vi "UHR-Fleezers Control (host) -Leonardo 04-2018 V3.vi"(0 "Tab Control":T5(tab)=enum."Trap Control (RF)") -> ()   [LabVIEW 2013] (continued)
              tunnel: w2124 -> [w2130]
              tunnel: w2122 -> [w2129]
              tunnel: w2121 -> [w2128]
              tunnel: w2120 -> [w2127]
              stop <- w2132 stop-if-true
              n1371 = event shown="[0] \"Pane\": Mouse Move" {
                selector: _ -> [_ _]
                dyn-events: _ -> [_ _]
                timeout: _ -> [_ _]
                tunnel: ["Force Manip Abort" w2196] -> w2132
                tunnel: w2131 -> [w2139 _]
                tunnel: w2130 -> [w2137 _]
                tunnel: w2129 -> [w2136 _]
                tunnel: w2128 -> [w2135 _]
                tunnel: w2127 -> [w2134 _]
                event Mouse Move {
                  n1372 = event-data() -> ("Time"=w2140:u32, "Coords"=w2141:T8)  [unwired: 3 out]
                  n1373 = Less?(x=w2140, y=w2139) -> (x < y?=w2138:bool)
                  n1374 = case "Makes sure old motion events prior to mouse click aren't used" shown="False" w2138 {
                    tunnel: w2141 -> [w2183 _]
                    tunnel: w2137 -> [w2184 _]
                    tunnel: w2136 -> [w2161 _]
                    tunnel: w2135 -> [w2157 _]
                    tunnel: w2134 -> [w2156 _]
                    frame False {
                      n1375 = Subtract(x=w2183, y=w2184) -> (x-y=w2182:T8)
                      "Coords" <- w2182
                      n1376 = local read "Y RF Frequency Limits (MHz)"() -> (w2142:T16)
                      n1377 = To Double Precision Float(number=w2182) -> (double precision float=w2181:cluster{"Horizontal":dbl, "Vertical":dbl})
                      n1378 = Multiply(x=cluster{"Horizontal":dbl, "Vertical":dbl} {"Horizontal"=-1.0, "Vertical"=1.0}, y="Manipulation Scaling") -> (x*y=w2177:cluster{"Horizontal":dbl, "Vertical":dbl})
                      n1379 = local read "X RF Frequency Limits (MHz)"() -> (w2143:T16)
                      n1380 = Multiply(x=w2181, y=w2177) -> (x*y=w2179:cluster{"Horizontal":dbl, "Vertical":dbl})
                      n1381 = Unbundle By Name(w2179) -> ("Horizontal"=w2174:dbl, "Vertical"=w2178:dbl)
                      n1382 = Unbundle By Name(w2142) -> ("Maximum"=w2145:dbl, "Minimum"=w2144:dbl)
                      n1383 = Boolean To (0,1)(Boolean="Manip. X?") -> (0, 1=w2172:i16)
                      n1384 = Boolean To (0,1)(Boolean="Manip. Y?") -> (0, 1=w2169:i16)
                      n1385 = local read "BD 1 Frequency 2 (MHz)"() -> (w2159:dbl)
                      n1386 = Multiply(x=w2178, y=w2169) -> (x*y=w2171:dbl)
                      n1387 = Multiply(x=w2172, y=w2174) -> (x*y=w2175:dbl)
                      n1388 = local read "BD 2 Frequency 2 (MHz)"() -> (w2158:dbl)
                      n1389 = Unbundle By Name(w2143) -> ("Maximum"=w2147:dbl, "Minimum"=w2146:dbl)
                      n1390 = Add(x=w2156, y=w2171) -> (x+y=w2149:dbl)
                      n1391 = Add(x=w2157, y=w2175) -> (x+y=w2151:dbl)
                      n1392 = In Range and Coerce(upper limit=w2147, x=w2151, lower limit=w2146) -> (coerced(x)=w2150:dbl)  [unwired: 1 out]
                      n1393 = In Range and Coerce(upper limit=w2145, x=w2149, lower limit=w2144) -> (coerced(x)=w2148:dbl)  [unwired: 1 out]
                      n1394 = Subtract(x=w2150, y=w2159) -> (x-y=w2168:dbl)
                      n1395 = Subtract(x=w2148, y=w2158) -> (x-y=w2167:dbl)
                      n1396 = Square(x=w2168) -> (x^2=w2166:dbl)
                      n1397 = Square(x=w2167) -> (x^2=w2165:dbl)
                      n1398 = Add(x=w2166, y=w2165) -> (x+y=w2164:dbl)
                      n1399 = Square Root(x=w2164) -> (sqrt(x)=w2160:dbl)
                      n1400 = In Range and Coerce(upper limit="Limit Max (MHz)", x=w2160, lower limit="Limit Min (MHz)") -> (In Range?=w2153:bool)  [unwired: 1 out]
                      n1401 = Not(x="Limits Enable") -> (.not. x?=w2152:bool)
                      n1402 = Or(x=w2153, y=w2152) -> (x .or. y?=w2154:bool)
                      n1403 = case shown="True" w2154 {
                        tunnel: w2161 -> [_ w2194]
                        tunnel: w2160 -> [_ w2185]
                        tunnel: w2150 -> [_ w2192]
                        tunnel: w2159 -> [_ w2191]
                        tunnel: w2148 -> [_ w2190]
                        tunnel: w2158 -> [_ w2189]
                        tunnel: w2143 -> [_ w2187]
                        tunnel: w2142 -> [_ w2186]
                        frame False {
                        }
                        frame True {
                          n1404 = local read "BD 1 Frequency 3 (MHz)"() -> (w2193:dbl)
                          n1405 = local read "BD 2 Frequency 3 (MHz)"() -> (w2188:dbl)
                          n1406 = local write "Trap Delta (MHz)"(w2185) -> ()
                          n1407 = property on="Initial delta (MHz)" class="DigNum (strict)"("Val(Sgnl)"=w2185) -> ()  [unwired: 2 in, 2 out]
                          n1408 = call "set RF board frequency - interlace.vi"("Board 2 Frequency Limits"=w2186, "Board 1 Frequency Limits"=w2187, "FPGA VI Reference In"=w2194, "Board 2 Frequency 3 (MHz)"=w2188, "Board 1 Frequency 3 (MHz)"=w2193, "Board 2 Frequency 2 (MHz)"=w2189, "Board 2 Frequency 1 (MHz)"=w2190, "Board 1 Frequency 2 (MHz)"=w2191, "Board 1 Frequency 1  (MHz)"=w2192) -> ()  [unwired: 1 in, 2 out]
                          n1409 = local write "BD 2 Frequency 1 (MHz)"(w2190) -> ()
                          n1410 = local write "BD 1 Frequency 1 (MHz)"(w2192) -> ()
                        }
                      }
                    }
                    frame True {
                    }
                  }
                }
                event Mouse Up {
                  n1411 = event-data() -> ("Button"=w2195:u16)  [unwired: 8 out]
                  n1412 = case shown="3" w2195 {
                    tunnel: [FALSE TRUE] -> w2196
                    frame 0, Default {
                    }
                    frame 3 {
                      n1413 = local write "Manipulating Trap"(FALSE ("Manipulating Trap")) -> ()
                    }
                  }
                }
              }
            }
          }
        }
      }
      event Mouse Move {
        n1414 = event-data() -> ()  [unwired: 6 out]
      }
    }
    n1415 = local read "Stop All"() -> (w2017:bool)
    n1416 = node-c288() -> ()  [unwired: 2 out]
  }
  n1417 = node-c288(w49) -> ()  [unwired: 1 out]
  n1418 = node-c288(w101) -> ()  [unwired: 1 out]
  n1419 = node-c288(w108) -> ()  [unwired: 1 out]
  n1420 = node-c288(i64 1 ("Period"), 1 ("Processor")) -> (w194:T25)  [unwired: 2 out]
  n1421 = timed-loop "Acquire Data" {
    tunnel: w57 -> [w2505]
    tunnel: w73 -> [w2504]
    tunnel: [w2535] -> w66
    tunnel: [w2529] -> w65
    timing: w194 -> [_]
    timing-out: [_] -> w193
    tunnel: w92 -> [w2351]
    stop <- "Stop All" stop-if-true
    (unwired) u32 0 ("Number of Elements")
    w2338 = "NI_ChannelName" ("name")
    n1422 = node-c288() -> ()  [unwired: 2 out]
    n1423 = First Call?() -> (First Call?: T/F=w2304:bool)
    n1424 = Or(x="Reset", y=w2304) -> (x .or. y?=w2305:bool)
    n1425 = local read "MCL Tracking"() -> (w2242:bool)
    n1426 = case "Reset data stream" shown="True" w2305 {
      tunnel: w2505 -> [w2655 w2663]
      tunnel: w2504 -> [w2654 w2662]
      tunnel: [w2655 w2657] -> w2240
      tunnel: [w2654 w2656] -> w2500
      frame False {
      }
      frame True {
        w2660 = TRUE ("AI to FIFO")
        n1427 = local write "Overflow (data lost)"(FALSE ("Overflow (data lost)")) -> ()
        n1428 = call "reset FPGA DMA.vi"("error in"=w2662, "FPGA VI Reference In"=w2663) -> ("error out"=w2658:errorcluster, "FPGA VI Reference Out"=w2659:T20)
        n1429 = xnode "Read/Write Control"("FPGA VI Reference In"=w2659, "error in"=w2658, "AI to FIFO"=w2660, "APD to FIFO"=w2660) -> ("FPGA VI Reference Out"=w2657:T20, "error out"=w2656:errorcluster)
      }
    }
    n1430 = Or(x="Start AOD Scan", y="Trap Raster Scan") -> (x .or. y?=w2458:bool)
    n1431 = case "Start AOM raster scan" shown="True" w2458 {
      tunnel: w2240 -> [w3396 w3407]
      tunnel: w2500 -> [w3395 w3406]
      tunnel: [w3396 w3400] -> w2239
      tunnel: [w3395 w3399] -> w2499
      frame False {
      }
      frame True {
        n1432 = case shown="True" "Restart DMA? (AOD)" {
          tunnel: [w3447 w3449] -> w3401
          tunnel: [w3446 w3448] -> w3402
          tunnel: w3407 -> [w3447 w3451]
          tunnel: w3406 -> [w3446 w3450]
          frame False {
          }
          frame True {
            n1433 = local write "Overflow (data lost)"(FALSE ("Overflow (data lost)")) -> ()
            n1434 = call "reset FPGA DMA.vi"("error in"=w3450, "FPGA VI Reference In"=w3451) -> ("error out"=w3448:errorcluster, "FPGA VI Reference Out"=w3449:T20)
          }
        }
        n1435 = local write "Trap Raster Scan"(FALSE ("Trap Raster Scan")) -> ()
        n1436 = case shown="True" "Move MCL Also?" {
          tunnel: w3402 -> [w3411 w3441]
          tunnel: w3401 -> [w3412 w3442]
          tunnel: [w3410 w3445] -> w3400
          tunnel: [w3409 w3444] -> w3399
          tunnel: "Raster to target force?" -> [w3408 w3414]
          frame False {
            w3413 = TRUE ("AI to FIFO")
            n1437 = xnode "Read/Write Control"("FPGA VI Reference In"=w3412, "error in"=w3411, "AI to FIFO"=w3413, "APD to FIFO"=w3413, "Start scan"=w3413, "Raster to target force"=w3408) -> ("FPGA VI Reference Out"=w3410:T20, "error out"=w3409:errorcluster)
          }
          frame True {
            w3438 = FALSE ("1D or 2D Scan?")
            w3443 = TRUE ("AI to FIFO")
            # "Count for MCL loop"
            # "N total cycles"
            # "N steps"
            # "V_int"
            n1438 = local read "Scan Range (nm)"() -> (w3420:dbl)
            n1439 = local read "Number of F/B Scans (AOD)"() -> (w3437:u16)
            n1440 = Sign(1:w3420) -> (0:w3419:dbl)
            n1441 = Compound Arithmetic op=MULTIPLY(w3420, "MCL Step Position Ratio", "MCL/AOM Scale Tweak") -> (w3424:dbl)
            n1442 = Negate(x=w3419) -> (-x=w3416:dbl)
            n1443 = Multiply(x=w3416, y="MCL Step Increment (V_int)") -> (x*y=w3418:dbl)
            n1444 = Divide(x=w3424, y="MCL X Cal (nm/V)") -> (x/y=w3430:dbl)
            n1445 = Multiply(x=32767.0 ("y"), y=w3430) -> (x*y=w3436:dbl)
            n1446 = local read "Total Counts (ticks)"() -> (w3421:u32)
            n1447 = local read "Cycles/step (AOD)"() -> (w3432:u64)
            n1448 = local read "Scan steps (AOD)"() -> (w3433:u64)
            n1449 = Divide(x=w3436, y=10.0) -> (x/y=w3429:dbl)
            n1450 = Divide(x=w3429, y="MCL Step Increment (V_int)") -> (x/y=w3427:dbl)
            n1451 = Absolute Value(x=w3427) -> (abs(x)=w3415:dbl)
            n1452 = Compound Arithmetic op=MULTIPLY(w3433, w3432, w3421) -> (w3428:u64)
            n1453 = local write "wait to reset values"(w3443) -> ()
            n1454 = local write "MCL Scanning"(w3443) -> ()
            n1455 = Divide(x=w3428, y=w3415) -> (x/y=w3425:dbl)
            "MCL Count" <- w3425
            n1456 = xnode "Read/Write Control"("FPGA VI Reference In"=w3442, "error in"=w3441, "Scan steps (MCL)"=w3415, "Number of scans (MCL)"=w3437, "Cycles per step (MCL)"=u64 1, "Scan freq.  increment (MCL)"=w3418, "1D or 2D Scan?"=w3438, "MCL Scan Axis"=w3438, "Cont. Scan (MCL)"=w3438, "MCL count"=w3425) -> ("FPGA VI Reference Out"=w3440:T20, "error out"=w3439:errorcluster)
            n1457 = xnode "Read/Write Control"("FPGA VI Reference In"=w3440, "error in"=w3439, "AI to FIFO"=w3443, "APD to FIFO"=w3443, "Start scan"=w3443, "Start scan (MCL)"=w3443, "Raster to target force"=w3414) -> ("FPGA VI Reference Out"=w3445:T20, "error out"=w3444:errorcluster)
          }
        }
        "Raster Scanning..." <- TRUE ("Scanning...")
      }
    }
    n1458 = And(x="Save scans", y=w2458) -> (x .and. y?=w2498:bool)
    n1459 = Compound Arithmetic op=OR("Start MCL Scan", "Confocal Image", "Confocal Linescan") -> (w2456:bool)
    n1460 = And(x="Save Data (MCL)", y=w2456) -> (x .and. y?=w2497:bool)
    n1461 = case "Start MCL raster scan" shown="True" w2456 {
      tunnel: w2239 -> [w2946 w2961]
      tunnel: w2499 -> [w2945 w2960]
      tunnel: [w2946 w2956] -> w2274
      tunnel: [w2945 w2955] -> w2273
      tunnel: [FALSE w2954] -> w2483
      tunnel: "Start MCL Scan" -> [_ w2949]
      tunnel: "Confocal Image" -> [_ w2948]
      tunnel: "Confocal Linescan" -> [_ _]
      frame False {
      }
      frame True {
        w2954 = TRUE
        n1462 = case shown="True" "Restart DMA? (MCL)" {
          tunnel: [w3006 w3008] -> w2959
          tunnel: [w3005 w3007] -> w2958
          tunnel: w2961 -> [w3006 w3011]
          tunnel: w2960 -> [w3005 w3010]
          frame False {
          }
          frame True {
            n1463 = call "reset FPGA DMA.vi"("error in"=w3010, "FPGA VI Reference In"=w3011) -> ("error out"=w3007:errorcluster, "FPGA VI Reference Out"=w3008:T20)
            n1464 = local write "Overflow (data lost)"(FALSE ("Overflow (data lost)")) -> ()
          }
        }
        n1465 = case shown="False" w2949 {
          selector: w2949 -> [_ w2965]
          tunnel: w2948 -> [w2964 _]
          tunnel: [w2964 w2965] -> w2947
          frame False {
            n1466 = property on="2D or 1D Scan" class="Bool (strict)"("Val(Sgnl)"=w2964) -> ()  [unwired: 2 in, 2 out]
            n1467 = property on="Confocal Image" class="Bool (strict)"("Value"=FALSE ("Start Confocal Map")) -> ()  [unwired: 2 in, 2 out]
          }
          frame True {
          }
        }
        n1468 = local write "MCL Scanning"(w2954) -> ()
        n1469 = local read "AO1"() -> (w2951:dbl)
        n1470 = local read "AO2"() -> (w2950:dbl)
        n1471 = case shown="True" "Center Scan" {
          tunnel: w2959 -> [w2972 w3004]
          tunnel: w2958 -> [w2971 w3003]
          tunnel: [w2970 w3002] -> w2956
          tunnel: [w2969 w3001] -> w2955
          tunnel: [w2967 w2988] -> w2953
          tunnel: [w2966 w2987] -> w2952
          tunnel: w2951 -> [w2967 w2993]
          tunnel: w2950 -> [w2966 w2996]
          tunnel: w2947 -> [_ _]
          frame False {
            w2968 = TRUE ("AI to FIFO")
            n1472 = xnode "Read/Write Control"("FPGA VI Reference In"=w2972, "error in"=w2971, "AI to FIFO"=w2968, "APD to FIFO"=w2968, "Start scan (MCL)"=w2968) -> ("FPGA VI Reference Out"=w2970:T20, "error out"=w2969:errorcluster)
          }
          frame True {
            w3000 = TRUE ("AI to FIFO")
            n1473 = local read "Scan steps (MCL)"() -> (w2979:u64)
            n1474 = local read "Scan lines (y)"() -> (w2975:u64)
            n1475 = local read "Fast Scan Dir"() -> (w2986:bool)
            n1476 = local read "Actual MCL Inc (V)"() -> (w2976:dbl)
            n1477 = Decrement(x=w2975) -> (x-1=w2974:u64)
            n1478 = Decrement(x=w2979) -> (x-1=w2978:u64)
            n1479 = Multiply(x=w2976, y=w2974) -> (x*y=w2973:dbl)
            n1480 = Divide(x=w2973, y=2.0) -> (x/y=w2983:dbl)
            n1481 = Multiply(x=w2976, y=w2978) -> (x*y=w2977:dbl)
            n1482 = Divide(x=w2977, y=2.0) -> (x/y=w2982:dbl)
            n1483 = Select(t=w2982, s=w2986, f=w2983) -> (s? t:f=w2981:dbl)
            n1484 = Select(t=w2983, s=w2986, f=w2982) -> (s? t:f=w2985:dbl)
            n1485 = Subtract(x=w2993, y=w2985) -> (x-y=w2984:dbl)
            n1486 = Subtract(x=w2996, y=w2981) -> (x-y=w2980:dbl)
            n1487 = local read "2D or 1D Scan"() -> (w2998:bool)
            n1488 = Not(x=w2986) -> (.not. x?=w2992:bool)
            n1489 = Not(x=w2998) -> (.not. x?=w2994:bool)
            n1490 = And(x=w2986, y=w2994) -> (x .and. y?=w2995:bool)
            n1491 = And(x=w2994, y=w2992) -> (x .and. y?=w2997:bool)
            n1492 = Select(t=w2996, s=w2997, f=w2980) -> (s? t:f=w2987:dbl)
            n1493 = Select(t=w2993, s=w2995, f=w2984) -> (s? t:f=w2988:dbl)
            n1494 = call "Volt to I16.vi"("Voltage In"=w2988) -> ("I16 Voltage Out"=w2991:i16)
            n1495 = call "Volt to I16.vi"("Voltage In"=w2987) -> ("I16 Voltage Out"=w2990:i16)
            n1496 = xnode "Read/Write Control"("FPGA VI Reference In"=w3004, "error in"=w3003, "AI to FIFO"=w3000, "APD to FIFO"=w3000, "Start scan (MCL)"=w3000, "AO1 (Y)"=w2991, "AO2 (X)"=w2990) -> ("FPGA VI Reference Out"=w3002:T20, "error out"=w3001:errorcluster)
          }
        }
        "Initial Y" <- w2953
        "Initial X" <- w2952
        "wait to reset values" <- w2954
      }
    }
    n1497 = local read "Trap Pos Elements/DMA read"() -> (w2347:u32)
    n1498 = local read "Trap AI Elements/DMA read"() -> (w2272:u32)
    n1499 = local read "APD Elements/DMA read"() -> (w2386:u32)
    n1500 = local read "Trap AI FIFO Depth"() -> (w2545:u32)
    n1501 = xnode "Invoke Method"("FPGA VI Reference In"=w2274, "error in"=w2273, "Number of Elements"=w2347, "Timeout (ms)"=-1) -> ("Data"=w2311:u16[], "Elements Remaining"=→"Trap Pos FIFO El Remaining":u32)  [unwired: 2 out]
    n1502 = xnode "Invoke Method"("FPGA VI Reference In"=w2274, "error in"=w2273, "Number of Elements"=w2272, "Timeout (ms)"=-1 ("Timeout")) -> ("FPGA VI Reference Out"=w2243:T20, "error out"=w2275:errorcluster, "Data"=w2271:i16[], "Elements Remaining"=w2276:u32)
    "Trap AI FIFO El. Rem." <- w2276
    n1503 = xnode "Get APD Data"("FPGA VI Reference In"=w2274, "error in"=w2273, "Number of Elements"=w2386, "Timeout (ms)"=-1) -> ("Data"=w2385:u32[], "Elements Remaining"=→"APD FIFO Elements Remaining":u32)  [unwired: 2 out]
    n1504 = Subtract(x=w2545, y=w2272) -> (x-y=w2544:u32)
    n1505 = Decimate 1D Array(w2311) -> (w2308:u16[], w2310:u16[], w2309:u16[])
    n1506 = Divide(x=w2276, y=w2544) -> (x/y=w2543:dbl)
    "Buffer Status" <- w2543
    n1507 = To Unsigned Long Integer(number=w2308) -> (unsigned 32bit integer=w2307:u32[])
    n1508 = Join Numbers(hi=w2310, lo=w2309) -> ((hi.lo)=w2306:u32[])
    n1509 = Equal?(x=w2543, y=1.0) -> (x = y?=w2541:bool)
    n1510 = Join Numbers(hi=w2307, lo=w2306) -> ((hi.lo)=w2300:u64[])
    n1511 = call "IR AOM word to freq - vec.vi"("Frequency Word In (double vec)"=w2300) -> ("Frequency Out"=w2346:dbl[])
    n1512 = case "Alert buffer overflow" shown="True" w2541 {
      frame False {
      }
      frame True {
        n1513 = call <vilib>:"Beep.vi"() -> ()  [unwired: 3 in, 9 out]
        "Overflow (data lost)" <- TRUE ("Overflow (data lost)")
      }
    }
    n1514 = Decimate 1D Array(w2346) -> (w2345:dbl[], w2344:dbl[])
    n1515 = Array Size(array=w2271) -> (size(s)=→"Waveform Chart":i32)
    n1516 = Build Array(w2345, w2344) -> (w2343:dbl[][])
    n1517 = local read "Trap Sets"() -> (w2418:u32)
    n1518 = case "Deinterlace trap data, average down PSD" shown="2" w2418 {
      tunnel: w2271 -> [w3041 w3106]
      tunnel: [w3038 w3103] -> w2411
      tunnel: [w3041 w3105] -> w2303
      tunnel: "Detector Type" -> [w3040 w3101]
      tunnel: [w3039 w3104] -> w2410
      tunnel: [w3037 w3102] -> w2516
      frame 1, Default {
        n1519 = Divide(x=w3041, y=3276.7) -> (x/y=w3042:dbl[])
        n1520 = Decimate 1D Array(w3042) -> (w3051:dbl[], w3050:dbl[], w3049:dbl[], w3048:dbl[], w3047:dbl[], w3046:dbl[], w3045:dbl[], w3044:dbl[])
        n1521 = case shown="\"IR-QPD + PSD + FB-QPD position\"" w3040 {
          tunnel: w3051 -> [w3075 w3100]
          tunnel: w3050 -> [w3074 w3099]
          tunnel: w3049 -> [w3059 w3077]
          tunnel: w3048 -> [w3060 w3087]
          tunnel: w3047 -> [w3073 w3098]
          tunnel: w3046 -> [w3072 w3097]
          tunnel: w3045 -> [w3056 w3078]
          tunnel: w3044 -> [w3055 w3076]
          tunnel: [w3054 w3084] -> w3039
          tunnel: [w3053 w3083] -> w3038
          tunnel: [w3052 w3082] -> w3037
          frame "IR-QPD + PSD + FB-QPD", Default {
            w3052 = 0  # Channel pattern
            n1522 = Divide(x=w3075, y=w3060) -> (x/y=w3062:dbl[])
            n1523 = Divide(x=w3074, y=w3060) -> (x/y=w3061:dbl[])
            n1524 = Divide(x=w3073, y=w3056) -> (x/y=w3058:dbl[])
            n1525 = Divide(x=w3072, y=w3055) -> (x/y=w3057:dbl[])
            n1526 = Build Array(w3062, w3061, w3060, w3059, w3058, w3057, w3056, w3055) -> (w3053:dbl[][])
            n1527 = Bundle("T1 Y", "T1 X", "T1 Sum", "FB Sum", "PSD Y", "PSD X", "PSD Y Sum", "PSD X Sum") -> (w3071:T42)  [unwired: 1 out]
            n1528 = Cluster To Array(cluster=w3071) -> (array=w3054:string[])
          }
          frame "IR-QPD + PSD + FB-QPD position" {
            w3082 = 3  # Channel pattern
            n1529 = Negate(x=w3078) -> (-x=w3079:dbl[])
            n1530 = Divide(x=w3100, y=w3087) -> (x/y=w3089:dbl[])
            n1531 = Divide(x=w3099, y=w3087) -> (x/y=w3088:dbl[])
            n1532 = Divide(x=w3098, y=w3078) -> (x/y=w3086:dbl[])
            n1533 = Divide(x=w3097, y=w3079) -> (x/y=w3085:dbl[])
            n1534 = Build Array(w3089, w3088, w3087, w3076, w3077, w3086, w3085, w3078) -> (w3083:dbl[][])
            n1535 = Bundle("T1 Y", "T1 X", "T1 Sum", "FB X", "FB Sum", "PSD Y", "PSD X", "PSD Y Sum") -> (w3096:T42)  [unwired: 1 out]
            n1536 = Cluster To Array(cluster=w3096) -> (array=w3084:string[])
          }
        }
      }
      frame 2 {
        n1537 = case shown="\"UCB Fleezers 052511\"" w3101 {
          tunnel: w3106 -> [w3168 w3235 w3274 w3374]
          tunnel: [w3107 w3227 w3270 w3305] -> w3105
          tunnel: [w3134 w3218 w3272 w3352] -> w3104
          tunnel: [w3133 w3182 w3263 w3319] -> w3103
          tunnel: [w3127 w3217 w3304 w3350] -> w3102
          frame "IR-QPD + PSD + FB-QPD", Default {
            w3127 = 1  # Channel pattern
            # "time average x2 the 4th signal and the 4 psd signals (detection laser)"
            # "deinterlace 3 signals from qpd"
            n1538 = Decimate 1D Array(w3168) -> (w3167:i16[], w3166:i16[], w3132:i16[], w3165:i16[], w3155:i16[], w3153:i16[], w3152:i16[], w3150:i16[])
            n1539 = call "downsample 1D array - double.vi"("Ave N"=2.0, "Array In"=w3155) -> ("Array Out"=w3154:dbl[])  [unwired: 1 out]
            n1540 = call "downsample 1D array - double.vi"("Ave N"=2.0, "Array In"=w3150) -> ("Array Out"=w3149:dbl[])  [unwired: 1 out]
            n1541 = call "downsample 1D array - double.vi"("Ave N"=2.0, "Array In"=w3152) -> ("Array Out"=w3151:dbl[])  [unwired: 1 out]
            n1542 = call "downsample 1D array - double.vi"("Ave N"=2.0, "Array In"=w3153) -> ("Array Out"=w3135:dbl[])  [unwired: 1 out]
            n1543 = Decimate 1D Array(w3167) -> (w3164:i16[], w3136:i16[])
            n1544 = Decimate 1D Array(w3166) -> (w3163:i16[], w3161:i16[])
            n1545 = Decimate 1D Array(w3165) -> (w3162:i16[], w3160:i16[])
            n1546 = Decimate 1D Array(w3132) -> (w3131:i16[], w3130:i16[])
            n1547 = Interleave 1D Arrays(w3164, w3163, w3162, w3136, w3161, w3160, w3131, w3130, w3154, w3135, w3151, w3149) -> (w3148:dbl[])
            n1548 = To Word Integer(number=w3148) -> (16bit integer=w3107:i16[])
            n1549 = Divide(x=w3148, y=3276.7) -> (x/y=w3147:dbl[])
            n1550 = Decimate 1D Array(w3147) -> (w3146:dbl[], w3145:dbl[], w3144:dbl[], w3143:dbl[], w3142:dbl[], w3141:dbl[], w3129:dbl[], w3128:dbl[], w3140:dbl[], w3139:dbl[], w3138:dbl[], w3137:dbl[])
            n1551 = Divide(x=w3146, y=w3144) -> (x/y=w3114:dbl[])
            n1552 = Divide(x=w3145, y=w3144) -> (x/y=w3113:dbl[])
            n1553 = Divide(x=w3143, y=w3141) -> (x/y=w3112:dbl[])
            n1554 = Divide(x=w3142, y=w3141) -> (x/y=w3111:dbl[])
            n1555 = Divide(x=w3140, y=w3138) -> (x/y=w3110:dbl[])
            n1556 = Divide(x=w3139, y=w3137) -> (x/y=w3109:dbl[])
            n1557 = Bundle("T1 Y", "T1 X", "T1 Sum", "T2 Y", "T2 X", "T2 Sum", "T1 FB Sum", "T2 FB Sum", "PSD Y", "PSD X", "PSD Y Sum", "PSD X Sum") -> (w3115:T43)  [unwired: 1 out]
            n1558 = Build Array(w3114, w3113, w3144, w3112, w3111, w3141, w3129, w3128, w3110, w3109, w3138, w3137) -> (w3133:dbl[][])
            n1559 = Cluster To Array(cluster=w3115) -> (array=w3134:string[])
          }
          frame "IR-QPD + PSD + FB-QPD X position" {
            w3217 = 2  # Channel pattern
            # "convert\nADC numbers\nto volts"
            # "time average x2 the 3 psd signals (detection laser)"
            # "deinterlace 3 signals from qpds"
            n1560 = Decimate 1D Array(w3235) -> (w3234:i16[], w3233:i16[], w3170:i16[], w3171:i16[], w3180:i16[], w3177:i16[], w3174:i16[], w3205:i16[])
            n1561 = Decimate 1D Array(w3234) -> (w3232:i16[], w3219:i16[])
            n1562 = call "downsample 1D array - I16.vi"("Ave N"=2.0, "Array In"=w3180) -> ("Array Out"=w3178:i16[])  [unwired: 1 in]
            n1563 = call "downsample 1D array - I16.vi"("Ave N"=2.0, "Array In"=w3177) -> ("Array Out"=w3175:i16[])  [unwired: 1 in]
            n1564 = Decimate 1D Array(w3233) -> (w3231:i16[], w3229:i16[])
            n1565 = Decimate 1D Array(w3171) -> (w3230:i16[], w3228:i16[])
            n1566 = Decimate 1D Array(w3205) -> (w3204:i16[], w3202:i16[])
            n1567 = Decimate 1D Array(w3170) -> (w3203:i16[], w3201:i16[])
            n1568 = call "downsample 1D array - I16.vi"("Ave N"=2.0, "Array In"=w3174) -> ("Array Out"=w3172:i16[])  [unwired: 1 in]
            n1569 = Interleave 1D Arrays(w3232, w3231, w3230, w3219, w3229, w3228, w3204, w3203, w3202, w3201, w3178, w3175, w3172) -> (w3227:i16[])
            n1570 = Divide(x=w3227, y=3276.7) -> (x/y=w3226:dbl[])
            n1571 = Decimate 1D Array(w3226) -> (w3225:dbl[], w3224:dbl[], w3223:dbl[], w3222:dbl[], w3221:dbl[], w3220:dbl[], w3193:dbl[], w3191:dbl[], w3190:dbl[], w3188:dbl[], w3187:dbl[], w3186:dbl[], w3183:dbl[])
            n1572 = Divide(x=w3225, y=w3223) -> (x/y=w3209:dbl[])
            n1573 = Divide(x=w3224, y=w3223) -> (x/y=w3208:dbl[])
            n1574 = Divide(x=w3222, y=w3220) -> (x/y=w3207:dbl[])
            n1575 = Divide(x=w3221, y=w3220) -> (x/y=w3206:dbl[])
            n1576 = Divide(x=w3193, y=w3191) -> (x/y=w3192:dbl[])
            n1577 = Divide(x=w3190, y=w3188) -> (x/y=w3189:dbl[])
            n1578 = Divide(x=w3187, y=w3183) -> (x/y=w3185:dbl[])
            n1579 = Negate(x=w3183) -> (-x=w3181:dbl[])
            n1580 = Divide(x=w3186, y=w3181) -> (x/y=w3184:dbl[])
            n1581 = Bundle("T1 Y", "T1 X", "T1 Sum", "T2 Y", "T2 X", "T2 Sum", "T1 FB X", "T1 FB Sum", "T2 FB X", "T2 FB Sum", "PSD Y", "PSD X", "PSD Y Sum") -> (w3210:T44)  [unwired: 1 out]
            n1582 = Build Array(w3209, w3208, w3223, w3207, w3206, w3220, w3192, w3191, w3189, w3188, w3185, w3184, w3183) -> (w3182:dbl[][])
            n1583 = Cluster To Array(cluster=w3210) -> (array=w3218:string[])
          }
          frame "UCB Fleezers 052511" {
            w3304 = 2  # Channel pattern
            n1584 = Select(t=i16 -1, s="Negate X signals", f=i16 1) -> (s? t:f=w3244:i16)
            n1585 = Decimate 1D Array(w3274) -> (w3245:i16[], w3246:i16[], w3257:i16[], w3273:i16[], w3242:i16[], w3240:i16[], w3238:i16[], w3254:i16[])
            n1586 = Multiply(x=w3244, y=w3246) -> (x*y=w3243:i16[])
            n1587 = Decimate 1D Array(w3245) -> (w3302:i16[], w3292:i16[])
            n1588 = Decimate 1D Array(w3243) -> (w3301:i16[], w3300:i16[])
            n1589 = Decimate 1D Array(w3257) -> (w3251:i16[], w3250:i16[])
            n1590 = Decimate 1D Array(w3273) -> (w3256:i16[], w3255:i16[])
            n1591 = Decimate 1D Array(w3240) -> (w3239:i16[])  [unwired: 1 out]
            n1592 = Decimate 1D Array(w3254) -> (w3253:i16[], w3252:i16[])
            n1593 = Decimate 1D Array(w3238) -> (w3237:i16[])  [unwired: 1 out]
            n1594 = Decimate 1D Array(w3242) -> (w3241:i16[])  [unwired: 1 out]
            n1595 = Interleave 1D Arrays(w3302, w3301, w3256, w3292, w3300, w3255, w3253, w3251, w3252, w3250, w3241, w3239, w3237) -> (w3270:i16[])
            n1596 = Divide(x=w3270, y=3276.7) -> (x/y=w3299:dbl[])
            n1597 = Decimate 1D Array(w3299) -> (w3298:dbl[], w3297:dbl[], w3296:dbl[], w3295:dbl[], w3294:dbl[], w3293:dbl[], w3269:dbl[], w3267:dbl[], w3266:dbl[], w3264:dbl[], w3262:dbl[], w3259:dbl[], w3260:dbl[])
            n1598 = Divide(x=w3298, y=w3296) -> (x/y=w3279:dbl[])
            n1599 = Divide(x=w3297, y=w3296) -> (x/y=w3278:dbl[])
            n1600 = Divide(x=w3295, y=w3293) -> (x/y=w3277:dbl[])
            n1601 = Divide(x=w3294, y=w3293) -> (x/y=w3276:dbl[])
            n1602 = Divide(x=w3269, y=w3267) -> (x/y=w3268:dbl[])
            n1603 = Divide(x=w3266, y=w3264) -> (x/y=w3265:dbl[])
            n1604 = Divide(x=w3262, y=w3260) -> (x/y=w3261:dbl[])
            n1605 = Divide(x=w3259, y=w3260) -> (x/y=w3258:dbl[])
            n1606 = Build Array(w3279, w3278, w3296, w3277, w3276, w3293, w3268, w3267, w3265, w3264, w3261, w3258, w3260) -> (w3263:dbl[][])
            n1607 = Bundle("T1 Y", "T1 X", "T1 Sum", "T2 Y", "T2 X", "T2 Sum", "T1 FB X", "T2 FB Sum", "T2 FB X", "T2 FB Sum", "PSD Y", "PSD X", "PSD Sum") -> (w3280:T44)  [unwired: 1 out]
            n1608 = Cluster To Array(cluster=w3280) -> (array=w3272:string[])
          }
          frame "IR-QPD + PSD + FB-QPD XY positions" {
            w3350 = 4  # Channel pattern
            # "time average x2 the 3 psd signals (detection laser)"
            # "deinterlace 3 signals from qpds"
            n1609 = Decimate 1D Array(w3374) -> (w3373:i16[], w3372:i16[], w3351:i16[], w3371:i16[], w3317:i16[], w3363:i16[], w3362:i16[], w3339:i16[])
            n1610 = Decimate 1D Array "QPD Y"(w3373) -> (w3370:i16[], w3353:i16[])
            n1611 = call "downsample 1D array - double.vi"("Ave N"=2.0, "Array In"=w3363) -> ("Array Out"=w3338:dbl[])  [unwired: 1 out]
            n1612 = call "downsample 1D array - double.vi"("Ave N"=2.0, "Array In"=w3362) -> ("Array Out"=w3337:dbl[])  [unwired: 1 out]
            n1613 = Decimate 1D Array "Feedback Sum"(w3351) -> (w3335:i16[], w3333:i16[])
            n1614 = Decimate 1D Array "Feedback Y"(w3317) -> (w3316:i16[], w3315:i16[])
            n1615 = Decimate 1D Array "Feedback X"(w3339) -> (w3336:i16[], w3334:i16[])
            n1616 = Decimate 1D Array "QPD Sum"(w3371) -> (w3368:i16[], w3366:i16[])
            n1617 = Decimate 1D Array "QPD X"(w3372) -> (w3369:i16[], w3367:i16[])
            n1618 = Interleave 1D Arrays(w3370, w3369, w3368, w3353, w3367, w3366, w3316, w3336, w3335, w3315, w3334, w3333, w3338, w3337) -> (w3361:dbl[])
            n1619 = To Word Integer(number=w3361) -> (16bit integer=w3305:i16[])
            n1620 = Divide(x=w3361, y=3276.7) -> (x/y=w3360:dbl[])
            n1621 = Decimate 1D Array(w3360) -> (w3359:dbl[], w3358:dbl[], w3357:dbl[], w3356:dbl[], w3355:dbl[], w3354:dbl[], w3312:dbl[], w3326:dbl[], w3310:dbl[], w3311:dbl[], w3324:dbl[], w3308:dbl[], w3322:dbl[], w3320:dbl[])
            n1622 = Divide(x=w3359, y=w3357) -> (x/y=w3343:dbl[])
            n1623 = Divide(x=w3358, y=w3357) -> (x/y=w3342:dbl[])
            n1624 = Divide(x=w3356, y=w3354) -> (x/y=w3341:dbl[])
            n1625 = Divide(x=w3355, y=w3354) -> (x/y=w3340:dbl[])
            n1626 = Divide(x=w3312, y=w3310) -> (x/y=w3309:dbl[])
            n1627 = Divide(x=w3326, y=w3310) -> (x/y=w3325:dbl[])
            n1628 = Divide(x=w3311, y=w3308) -> (x/y=w3307:dbl[])
            n1629 = Divide(x=w3324, y=w3308) -> (x/y=w3323:dbl[])
            n1630 = Negate(x=w3320) -> (-x=w3318:dbl[])
            n1631 = Divide(x=w3322, y=w3318) -> (x/y=w3321:dbl[])
            n1632 = Bundle("T1 Y", "T1 X", "T1 Sum", "T2 Y", "T2 X", "T2 Sum", "T1 FB Y", "T1 FB X", "T1 FB Sum", "T2 FB Y", "T2 FB X", "T2 FB Sum", "PSD X", "PSD Y Sum") -> (w3306:T45)  [unwired: 1 out]
            n1633 = Build Array(w3343, w3342, w3357, w3341, w3340, w3354, w3309, w3325, w3310, w3307, w3323, w3308, w3321, w3320) -> (w3319:dbl[][])
            n1634 = Cluster To Array(cluster=w3306) -> (array=w3352:string[])
          }
        }
      }
    }
    "AI labels" <- w2410
    n1635 = xnode "Read/Write Control"("FPGA VI Reference In"=w2243) -> ("FPGA VI Reference Out"=w2236:T20, "BD1 Frequency Out 1"=w2257:u64)  [unwired: 1 in, 1 out]
    n1636 = local read "BD 1 Frequency 2 (MHz)"() -> (w2248:dbl)
    n1637 = To Double Precision Float(number=w2257) -> (double precision float=w2254:dbl)
    n1638 = Multiply(x=49125000.0, y=6.0) -> (x*y=w2253:dbl)
    n1639 = Multiply(x=w2254, y=w2253) -> (x*y=w2251:dbl)
    n1640 = Scale By Power Of 2(n=-48, x=w2251) -> (x*2^n=w2250:dbl)
    n1641 = local read "Dynamic Force FB"() -> (w2247:bool)
    n1642 = local read "Trap Pos. FB ON"() -> (w2246:bool)
    n1643 = Divide(x=w2250, y=1000000.0) -> (x/y=w2241:dbl)
    n1644 = case shown="True" w2242 {
      tunnel: w2241 -> [_ w2632]
      tunnel: w2239 -> [_ w2619]
      frame False {
      }
      frame True {
        n1645 = local read "AOM X Cal (nm/MHz)"() -> (w2629:dbl)
        n1646 = local read "Zero T1 position"() -> (w2631:dbl)
        n1647 = Subtract(x=w2632, y=w2631) -> (x-y=w2630:dbl)
        n1648 = Multiply(x=w2630, y=w2629) -> (x*y=w2628:dbl)
        n1649 = local read "MCL X Cal (nm/V)"() -> (w2625:dbl)
        n1650 = Multiply(x=w2628, y="Tracking factor") -> (x*y=w2626:dbl)
        n1651 = local read "Zero MCL x position"() -> (w2624:dbl)
        n1652 = Divide(x=w2626, y=w2625) -> (x/y=w2623:dbl)
        n1653 = Add(x=w2624, y=w2623) -> (x+y=w2616:dbl)
        "Current MCL (V)" <- w2616
        n1654 = Multiply(x=w2616, y=32767.0) -> (x*y=w2620:dbl)
        n1655 = Divide(x=w2620, y=10.0) -> (x/y=w2617:dbl)
        n1656 = To Word Integer(number=w2617) -> (16bit integer=w2618:i16)
        n1657 = xnode "Read/Write Control"("FPGA VI Reference In"=w2619, "AO2 (X)"=w2618) -> ()  [unwired: 1 in, 2 out]
      }
    }
    n1658 = Subtract(x=w2248, y=w2241) -> (x-y=w2237:dbl)
    "Current deltaFreq" <- w2237
    n1659 = Compound Arithmetic op=AND(w2247, w2246, "Real time offset \ncorrection for setpoint") -> (w2244:bool)
    n1660 = case shown="True" w2244 {
      tunnel: w2237 -> [_ w2635]
      tunnel: w2236 -> [_ w2634]
      frame False {
      }
      frame True {
        n1661 = local read "T1 kappa_x (pN/nm)"() -> (w2643:dbl)
        n1662 = local read "T1 alpha_x (nm/V)"() -> (w2644:dbl)
        n1663 = local read "Negate offset difference"() -> (w2645:bool)
        n1664 = local read "Offset file step size"() -> (w2653:dbl)
        n1665 = Multiply(x="Target Force (pN)", y=2.0) -> (x*y=w2641:dbl)
        n1666 = local read "Setpoint offset\nCorrection values"() -> (w2650:dbl[])
        n1667 = Divide(x=w2635, y=w2653) -> (x/y=w2652:dbl)
        n1668 = Select(t=-1, s=w2645, f=1) -> (s? t:f=w2646:i32)
        n1669 = To Long Integer(number=w2652) -> (32bit integer=w2651:i32)
        n1670 = Multiply(x=w2644, y=w2643) -> (x*y=w2640:dbl)
        n1671 = Divide(x=w2641, y=w2640) -> (x/y=w2639:dbl)
        n1672 = Index Array(array=w2650, index=w2651) -> (element=w2649:dbl)
        n1673 = Multiply(x=w2646, y=w2649) -> (x*y=w2638:dbl)
        n1674 = Add(x=w2639, y=w2638) -> (x+y=w2637:dbl)
        n1675 = To Fixed-Point(number=w2637) -> (fixed-point=w2633:fxp<+/-,16,1>)  [unwired: 1 in]
        "Actual setpoint" <- w2633
        n1676 = xnode "Read/Write Control"("FPGA VI Reference In"=w2634, "Trap Pos. FB SP"=w2633) -> ()  [unwired: 1 in, 2 out]
      }
    }
    n1677 = case shown="True" "Take full offset\n data for display" {
      tunnel: [w2602 w2608] -> w2435
      tunnel: [w2601 w2607] -> w2433
      tunnel: w2237 -> [_ w2614]
      frame False {
        n1678 = Divide(x="T2 offset_x (mV)", y=1000.0) -> (x/y=w2601:dbl)
        n1679 = Divide(x="T1 offset_x (mV)", y=1000.0) -> (x/y=w2602:dbl)
      }
      frame True {
        n1680 = local read "Offset Values"() -> (w2615:T14)
        n1681 = local read "Offset file step size"() -> (w2613:dbl)
        n1682 = Unbundle By Name(w2615) -> ("Trap 1X offset"=w2610:dbl[], "Trap 2X offset"=w2609:dbl[])
        n1683 = Divide(x=w2614, y=w2613) -> (x/y=w2612:dbl)
        n1684 = To Long Integer(number=w2612) -> (32bit integer=w2611:i32)
        n1685 = Index Array(array=w2610, index=w2611) -> (element=w2608:dbl)
        n1686 = Index Array(array=w2609, index=w2611) -> (element=w2607:dbl)
      }
    }
    n1687 = Decimate 1D Array(w2385) -> (w2408:u32[], w2353:u32[])
    n1688 = local read "DMA Update Period (s)"() -> (w2419:dbl)
    n1689 = local read "BD 1 Frequency 2 (MHz)"() -> (w2295:dbl)
    n1690 = local read "BD 1 Frequency 1 (MHz)"() -> (w2296:dbl)
    n1691 = Build Array(w2408, w2353) -> (w2480:u32[][])
    n1692 = local read "Data Period (s)"() -> (w2398:dbl)
    n1693 = Decimate 1D Array(w2303) -> (w2326:i16[], w2325:i16[], w2323:i16[], w2322:i16[])  [unwired: 9 out]
    n1694 = To Double Precision Float(number=w2480) -> (double precision float=w2481:dbl[][])
    n1695 = local read "APD Integration Time (s)"() -> (w2366:dbl)
    n1696 = Divide(x=w2326, y=w2325) -> (x/y=w2327:dbl[])
    n1697 = Divide(x=w2323, y=w2322) -> (x/y=w2324:dbl[])
    n1698 = feedback #1(0.0) -> (w2340:dbl)
    n1699 = Add(x=w2419, y=w2340) -> (x+y=w2518:dbl)
    n1700 = feedback-in #1(w2518) -> ()
    n1701 = local read "AOM X Cal (nm/MHz)"() -> (w2293:dbl)
    n1702 = To Time Stamp(1:w2340) -> (0:w2339:timestamp)
    n1703 = Split 1D Array(array=w2327, index="N El. to Ave.") -> (second subarray=w2330:dbl[])  [unwired: 1 out]
    n1704 = Split 1D Array(array=w2324, index="N El. to Ave.") -> (second subarray=w2329:dbl[])  [unwired: 1 out]
    n1705 = local read "Trap X AI1 (DMA)"() -> (w2328:T13)
    n1706 = Multiply(x=w2398, y="Trap Disp. Downsample") -> (x*y=w2341:dbl)
    "Display Period (s)" <- w2341
    n1707 = Bundle("BD 1 Frequency 1 (MHz)"=w2296, "BD 1 Frequency 2 (MHz)"=w2295) -> (w2297:T46)  [unwired: 1 out]
    n1708 = for "Trap AI" {
      tunnel: [w3036] -> w2512 mode=indexing
      tunnel: w2339 -> [w3026]
      tunnel: "Trap Disp. Downsample" -> [w3034]
      tunnel: w2411 -> [w3032] mode=indexing
      tunnel: w2398 -> [w3031]
      tunnel: w2410 -> [w3030] mode=indexing
      tunnel: w2338 -> [w3029]
      tunnel: [w3028] -> w2377 mode=indexing
      tunnel: w2341 -> [w3027]
      n1709 = Bundle By Name("Y"=w3032, "dt"=w3031) -> (w3033:waveform(dbl))  [unwired: 1 out]
      n1710 = Set Waveform Attribute(5:w3030, 6:w3029, 7:w3033) -> (3:w3028:waveform(dbl))  [unwired: 1 in, 2 out]
      n1711 = call "downsample 1D array - double.vi"("Ave N"=w3034, "Array In"=w3032) -> ("Array Out"=w3035:dbl[])  [unwired: 1 out]
      n1712 = Bundle By Name(cluster=w3028, "t0"=w3026, "Y"=w3035, "dt"=w3027) -> (w3036:waveform(dbl))
    }
    n1713 = call-poly <vilib>:"Mean.vi"("X"=w2329) -> ("mean"=w2317:dbl)  [unwired: 1 out]
    n1714 = call-poly <vilib>:"Mean.vi"("X"=w2330) -> ("mean"=w2318:dbl)  [unwired: 1 out]
    n1715 = Cluster To Array(cluster=w2297) -> (array=w2294:dbl[])
    n1716 = Reciprocal(x=w2341) -> (1/x=→"Trap Disp. Freq. (Hz)":dbl)
    n1717 = local read "Data points/scans (MCL)"() -> (w2492:dbl)
    n1718 = To Fixed-Point(number=w2317) -> (fixed-point=w2315:fxp<+/-,16,1>)  [unwired: 1 in]
    n1719 = To Fixed-Point(number=w2318) -> (fixed-point=w2316:fxp<+/-,16,1>)  [unwired: 1 in]
    n1720 = Bundle("Trap 1 Pos.", "Trap 2 Pos.") -> (w2337:cluster{string, string})  [unwired: 1 out]
    n1721 = Bundle By Name(cluster=w2328, "Set 1"=w2316, "Set 2"=w2315) -> (→"Trap X AI1 (DMA)":T13)
    n1722 = Cluster To Array(cluster=w2337) -> (array=w2334:string[])
    n1723 = for "Trap Position" {
      tunnel: w2343 -> [w2676] mode=indexing
      tunnel: "Trap Disp. Downsample" -> [w2675]
      tunnel: w2341 -> [w2673]
      tunnel: w2339 -> [w2672]
      tunnel: w2338 -> [w2670]
      tunnel: w2334 -> [w2669] mode=indexing
      tunnel: [w2668] -> w2292 mode=indexing
      tunnel: w2294 -> [w2666] mode=indexing
      tunnel: w2293 -> [w2664]
      n1724 = call "downsample 1D array - double.vi"("Ave N"=w2675, "Array In"=w2676) -> ("Array Out"=w2674:dbl[])  [unwired: 1 out]
      n1725 = Subtract(x=w2674, y=w2666) -> (x-y=w2667:dbl[])
      n1726 = Multiply(x=w2664, y=w2667) -> (x*y=w2665:dbl[])
      n1727 = Bundle By Name("Y"=w2665, "dt"=w2673, "t0"=w2672) -> (w2671:waveform(dbl))  [unwired: 1 out]
      n1728 = Set Waveform Attribute(5:w2669, 6:w2670, 7:w2671) -> (3:w2668:waveform(dbl))  [unwired: 1 in, 2 out]
    }
    "Trap Positions" <- w2292
    n1729 = Bundle("APD 1", "APD 2") -> (w2511:cluster{string, string})  [unwired: 1 out]
    n1730 = Cluster To Array(cluster=w2511) -> (array=w2508:string[])
    n1731 = for "APD" {
      tunnel: w2481 -> [w3015] mode=indexing
      tunnel: w2366 -> [w3023]
      tunnel: [w3019] -> w2373 mode=indexing
      tunnel: "APD Disp. Scale" -> [w3020]
      tunnel: w2338 -> [w3018]
      tunnel: w2508 -> [w3017] mode=indexing
      tunnel: "APD Disp. Downsample" -> [w3013]
      tunnel: [w3016] -> w2507
      tunnel: w2339 -> [w3012]
      n1732 = call "integrate 1D array interval - double.vi"("Ave N"=w3013, "Array In"=w3015) -> ("Array Out"=w3014:dbl[])  [unwired: 1 out]
      n1733 = Multiply(x=w3023, y=w3013) -> (x*y=w3016:dbl)
      n1734 = Divide(x=w3014, y=w3020) -> (x/y=w3021:dbl[])
      n1735 = Bundle By Name("t0"=w3012, "Y"=w3021, "dt"=w3016) -> (w3022:waveform(dbl))  [unwired: 1 out]
      n1736 = Set Waveform Attribute(5:w3017, 6:w3018, 7:w3022) -> (3:w3019:waveform(dbl))  [unwired: 1 in, 2 out]
    }
    "APD Display Period (s)" <- w2507
    n1737 = Reciprocal(x=w2507) -> (1/x=→"APD Display Freq. (Hz)":dbl)
    n1738 = local read "Display Period (s)"() -> (w2397:dbl)
    n1739 = Increment(x=w2492) -> (x+1=w2493:dbl)
    n1740 = Index Array(array=w2292, index=0) -> (element=w2290:waveform(dbl))
    n1741 = To Double Precision Float(number=w2408) -> (double precision float=w2407:dbl[])
    n1742 = feedback #2(w2493) -> (w2496:dbl)
    n1743 = Select(t=0, s=w2483, f=w2496) -> (s? t:f=w2489:dbl)
    n1744 = Array Size(array=w2407) -> (size(s)=w2495:i32)
    n1745 = Add(x=w2495, y=w2489) -> (x+y=w2490:dbl)
    n1746 = Unbundle By Name(w2290) -> ("Y"=w2288:dbl[])
    n1747 = feedback #3(w2408) -> (w2479:u32[])
    n1748 = Build Array (concatenate)(w2479, w2408) -> (w2476:u32[])
    n1749 = feedback #4(w2353) -> (w2372:u32[])
    n1750 = Divide(x="Bead Sep. Int. Time (s)", y=w2397) -> (x/y=w2286:dbl)
    n1751 = Build Array (concatenate)(w2372, w2353) -> (w2371:u32[])
    n1752 = Greater?(x=w2490, y=w2492) -> (0:w2491:bool)
    n1753 = feedback #5(w2288) -> (w2289:dbl[])
    n1754 = Build Array (concatenate)(w2288, w2289) -> (w2287:dbl[])
    n1755 = Select(t=w2489, s=w2491, f=w2490) -> (s? t:f=w2488:dbl)
    n1756 = feedback-in #2(w2488) -> ()
    n1757 = Array Size(array=w2476) -> (size(s)=w2473:i32)
    n1758 = Array Size(array=w2408) -> (size(s)=w2475:i32)
    n1759 = local read "MCL Scanning"() -> (w2486:bool)
    n1760 = local read "APD Integration Time (s)"() -> (w2380:dbl)
    n1761 = Build Array (concatenate)(w2373, w2512) -> (w2375:waveform(dbl)[])
    "All Signals" <- w2375
    n1762 = Split 1D Array(array=w2287, index=w2286) -> (first subarray=w2280:dbl[])  [unwired: 1 out]
    n1763 = feedback-in #5(w2280) -> ()
    n1764 = Multiply(x=w2475, y="APD Ave N") -> (x*y=w2474:dbl)
    n1765 = Greater?(x=w2473, y=w2474) -> (0:w2477:bool)
    n1766 = Not(x=w2491) -> (.not. x?=w2485:bool)
    n1767 = To Double Precision Float(number=w2353) -> (double precision float=w2352:dbl[])
    n1768 = call-poly <vilib>:"Mean.vi"("X"=w2280) -> ("mean"=w2279:dbl)  [unwired: 1 out]
    "Mean T1 Position (nm)" <- w2279
    n1769 = Subtract(x=w2280, y=w2279) -> (x-y=w2285:dbl[])
    n1770 = Square(x=w2285) -> (x^2=w2284:dbl[])
    n1771 = And(x=w2485, y=w2486) -> (x .and. y?=w2487:bool)
    n1772 = call-poly <vilib>:"Mean.vi"("X"=w2284) -> ("mean"=w2283:dbl)  [unwired: 1 out]
    n1773 = case shown="True" w2477 {
      tunnel: w2476 -> [w2796 w2803]
      tunnel: [w2796 w2801] -> w2424
      tunnel: w2474 -> [_ w2798]
      tunnel: w2473 -> [_ w2802]
      tunnel: w2371 -> [w2795 w2800]
      tunnel: [w2795 w2797] -> w2368
      frame False {
      }
      frame True {
        n1774 = Subtract(x=w2802, y=w2798) -> (x-y=w2799:dbl)
        n1775 = Array Subset(array=w2803, index=w2799, length=w2798) -> (w2801:u32[])
        n1776 = Array Subset(array=w2800, index=w2799, length=w2798) -> (w2797:u32[])
      }
    }
    n1777 = feedback-in #3(w2424) -> ()
    n1778 = feedback-in #4(w2368) -> ()
    n1779 = Or(x=w2487, y=w2483) -> (x .or. y?=w2484:bool)
    n1780 = Square Root(x=w2283) -> (sqrt(x)=w2282:dbl)
    n1781 = Equal?(x="Tab Control 6", y=T36."High Res Display") -> (x = y?=w2414:bool)
    n1782 = Multiply(x="APD Disp. Scale", y=w2373) -> (x*y=w2382:waveform(dbl)[])
    n1783 = Multiply(x="APD Disp. Downsample", y=w2380) -> (x*y=w2378:dbl)
    n1784 = Multiply(x=10.0, y=w2282) -> (x*y=→"Trap 1 Position RMS (A)":dbl)
    n1785 = Divide(x=w2382, y=w2378) -> (x/y=w2350:waveform(dbl)[])
    n1786 = Index Array(array=w2350, index=0) -> (element=w2360:waveform(dbl))
    n1787 = case "For computing FFTs for display" shown="True" "Compute FFT" {
      tunnel: w2377 -> [_ w3480]
      frame False {
      }
      frame True {
        n1788 = Build Array("FFT 1 Choice 1", "FFT 1 Choice 2", "FFT 2 Choice 1", "FFT 2 Choice 2") -> (w3473:u16[])
        n1789 = Array Size(array=w3480) -> (size(s)=w3479:i32)
        n1790 = feedback-in #6(w3473) -> ()
        n1791 = feedback #6(u16[] [100, 100, 100, 100]) -> (w3474:u16[])
        n1792 = feedback-in #7("# Spectra to Ave.") -> ()
        n1793 = feedback #7("# Spectra to Ave.") -> (w3471:dbl)
        n1794 = Not Equal?(x="# Spectra to Ave.", y=w3471) -> (x != y?=w3470:bool)
        n1795 = Not Equal?(x=w3473, y=w3474) -> (x != y?=w3472:bool)
        n1796 = feedback #8(1.0) -> (w3457:dbl)
        n1797 = Compound Arithmetic op=OR("Reset FFT", w3472, w3470) -> (w3455:bool)
        n1798 = Select(t=1.0, s=w3455, f=w3457) -> (s? t:f=w3459:dbl)
        n1799 = Greater?(x=w3459, y="# Spectra to Ave.") -> (0:w3478:bool)
        n1800 = Increment(x=w3459) -> (x+1=w3458:dbl)
        n1801 = feedback-in #8(w3458) -> ()
        n1802 = local read "DMA Update Period (s)"() -> (w3453:dbl)
        n1803 = Multiply(x="# Spectra to Ave.", y=w3453) -> (x*y=→"Ave. Time (s)":dbl)
        n1804 = Build Array(cluster{"f0":dbl, "df":dbl, "magnitude":dbl[]} {"f0"=0.0, "df"=0.0, "magnitude"=[]} ("PSD")) -> (w3462:cluster{"f0":dbl, "df":dbl, "magnitude":dbl[]}[])
        n1805 = Build Array(w3462, w3462, w3462, w3462) -> (w3464:T47)
        n1806 = feedback #9(w3464) -> (w3469:T47)
        n1807 = for {
          N: 4 -> [_]
          tunnel: w3473 -> [w3502] mode=indexing
          tunnel: w3480 -> [w3503]
          tunnel: w3479 -> [w3505]
          tunnel: w3455 -> [w3498]
          tunnel: w3478 -> [w3497]
          tunnel: "# Spectra to Ave." -> [w3496]
          tunnel: [w3495] -> w3468 mode=indexing
          tunnel: w3469 -> [w3500] mode=indexing
          tunnel: [w3499] -> w3456 mode=indexing
          tunnel: w3459 -> [w3494]
          n1808 = Less?(x=w3502, y=w3505) -> (x < y?=w3504:bool)
          n1809 = Index Array(array=w3503, index=w3502) -> (element=w3501:waveform(dbl))
          n1810 = case shown="True" w3504 {
            tunnel: w3501 -> [_ w3522]
            tunnel: w3500 -> [w3507 w3520]
            tunnel: [w3507 w3508] -> w3499
            tunnel: w3498 -> [_ w3519]
            tunnel: w3497 -> [_ w3512]
            tunnel: w3496 -> [_ w3511]
            tunnel: [cluster{"f0":dbl, "df":dbl, "magnitude":dbl[]} {"f0"=0.0, "df"=0.0, "magnitude"=[]} ("PSD") w3513] -> w3495
            tunnel: w3494 -> [_ w3510]
            frame False {
            }
            frame True {
              n1811 = call <vilib>:"Std Deviation and Variance.vi"("X"=w3522) -> ("mean"=w3523:dbl)  [unwired: 1 in, 2 out]
              n1812 = Subtract(x=w3522, y=w3523) -> (x-y=w3521:waveform(dbl))
              n1813 = xnode "Spectral Measurements"("Signals"=w3521) -> ("PSD"=w3515:cluster{"f0":dbl, "df":dbl, "magnitude":dbl[]})  [unwired: 1 in, 1 out]
              n1814 = case shown="False" w3519 {
                tunnel: w3520 -> [w3532 _]
                tunnel: [w3528 w3537] -> w3508
                tunnel: w3515 -> [w3531 w3538]
                tunnel: w3512 -> [w3530 _]
                frame False {
                  n1815 = Build Array (concatenate)(w3532, w3531) -> (w3529:cluster{"f0":dbl, "df":dbl, "magnitude":dbl[]}[])
                  n1816 = case shown="True" w3530 {
                    tunnel: w3529 -> [w3533 w3536]
                    tunnel: [w3533 w3534] -> w3528
                    frame False {
                    }
                    frame True {
                      n1817 = Delete From Array(array=w3536, index=0) -> (array with subset deleted=w3534:cluster{"f0":dbl, "df":dbl, "magnitude":dbl[]}[])  [unwired: 1 in, 1 out]
                    }
                  }
                }
                frame True {
                  n1818 = Build Array(w3538) -> (w3537:cluster{"f0":dbl, "df":dbl, "magnitude":dbl[]}[])
                }
              }
              n1819 = for {
                tunnel: w3508 -> [w3527] mode=indexing
                tunnel: [w3526] -> w3518 mode=indexing
                workers-P: _ -> [_]
                n1820 = Unbundle By Name(w3527) -> ("magnitude"=w3526:dbl[])
              }
              n1821 = Transpose 2D Array(2D array=w3518) -> (transposed array=w3517:dbl[][])
              n1822 = for {
                tunnel: w3517 -> [w3525] mode=indexing
                tunnel: [w3524] -> w3516 mode=indexing
                workers-P: _ -> [_]
                n1823 = Add Array Elements(numeric array=w3525) -> (sum=w3524:dbl)
              }
              n1824 = Select(t=w3511, s=w3512, f=w3510) -> (s? t:f=w3509:dbl)
              n1825 = Divide(x=w3516, y=w3509) -> (x/y=w3514:dbl[])
              n1826 = Bundle By Name(cluster=w3515, "magnitude"=w3514) -> (w3513:cluster{"f0":dbl, "df":dbl, "magnitude":dbl[]})
            }
          }
        }
        n1827 = case shown="True" w3455 {
          tunnel: w3456 -> [w3487 w3493]
          tunnel: [w3487 w3488] -> w3454
          frame False {
          }
          frame True {
            n1828 = Array Subset(array=w3493, index (row)=0 ("index"), length (row)=4 ("length"), index (col)=0 ("index"), length (col)=1 ("length")) -> (w3488:T47)
          }
        }
        n1829 = feedback-in #9(w3454) -> ()
        n1830 = Split 1D Array(array=w3468, index=2) -> (first subarray=→"FFT 1":cluster{"f0":dbl, "df":dbl, "magnitude":dbl[]}[], second subarray=→"FFT 2":cluster{"f0":dbl, "df":dbl, "magnitude":dbl[]}[])
      }
    }
    n1831 = Index Array(array=w2350, index=1) -> (element=w2358:waveform(dbl))
    n1832 = case "For displaying the high resolution display (no downsampling)" shown="True" w2414 {
      tunnel: w2377 -> [_ w2696]
      frame False {
      }
      frame True {
        n1833 = Index Array(array=w2696, index="High Res. Display") -> (element=w2697:waveform(dbl))
        n1834 = call <vilib>:"Std Deviation and Variance.vi"("X"=w2697) -> ("mean"=w2704:dbl, "standard deviation"=w2709:dbl)  [unwired: 1 in, 1 out]
        "Mean Intensity" <- w2704
        "Sigma" <- w2709
        n1835 = Subtract(x=w2697, y=w2704) -> (x-y=w2703:waveform(dbl))
        n1836 = Select(t=w2703, s="Subtract mean", f=w2697) -> (s? t:f=→"1 Channel":waveform(dbl))
        n1837 = Divide(x=w2709, y=w2704) -> (x/y=→"Sigma/Mean":dbl)
        n1838 = feedback #10(1) -> (w2698:i32)
        n1839 = Greater Or Equal?(x=w2698, y="Slow mean N ave.") -> (x >= y?=w2711:bool)
        n1840 = Increment(x=w2698) -> (x+1=w2713:i32)
        n1841 = Select(t=1, s=w2711, f=w2713) -> (s? t:f=w2700:i32)
        n1842 = feedback-in #10(w2700) -> ()
        n1843 = feedback #11() -> (w2701:waveform(dbl))  [unwired: 1 out]
        n1844 = case shown="Default" w2698 {
          tunnel: [w2716 w2719] -> w2702
          tunnel: w2701 -> [w2718 _]
          tunnel: w2697 -> [w2717 w2719]
          frame Default {
            n1845 = call-poly <vilib>:"Append Waveforms.vi"("waveform B"=w2717, "waveform A"=w2718) -> ("waveform out"=w2716:waveform(dbl))  [unwired: 1 in, 8 out]
          }
          frame 1 {
          }
        }
        n1846 = feedback-in #11(w2702) -> ()
        n1847 = case shown="True" w2711 {
          tunnel: w2702 -> [_ w2715]
          frame False {
          }
          frame True {
            n1848 = call-poly <vilib>:"Mean.vi"("X"=w2715) -> ("mean"=→"Slow mean":dbl)  [unwired: 1 out]
          }
        }
      }
    }
    n1849 = case "For plotting results of scanning MCL" shown="True" w2484 {
      tunnel: w2483 -> [_ w2836]
      tunnel: w2407 -> [_ w2932]
      tunnel: w2492 -> [_ _]
      tunnel: w2377 -> [_ w2906]
